vi "Catagorize VI.vi"(8 "error in (no error)":errorcluster {"code" format="Error %.0f"}, 10 "VI Reference":refnum<vi>, 11 "VIDoc Parser In":refnum<class "VIDoc Parser.lvclass">) -> (0 "error out":errorcluster {"code" format="Error %.0f"}, 3 "VIDoc Parser Out":refnum<class "VIDoc Parser.lvclass">)   [LabVIEW 2023, in "VIDoc Parsing.lvlib" / "VIDoc Parser.lvclass"]
uses:
  VIDoc Parser.lvclass
  VIDoc Parser.lvclass/VIDoc Parser.ctl
  <vilib>/Utility/lvfile.llb/NI_FileType.lvlib
  <vilib>/Utility/miscctls.llb/LVMapReplaceAction.ctl
  GUI Documentation/GUI Documentation.lvclass
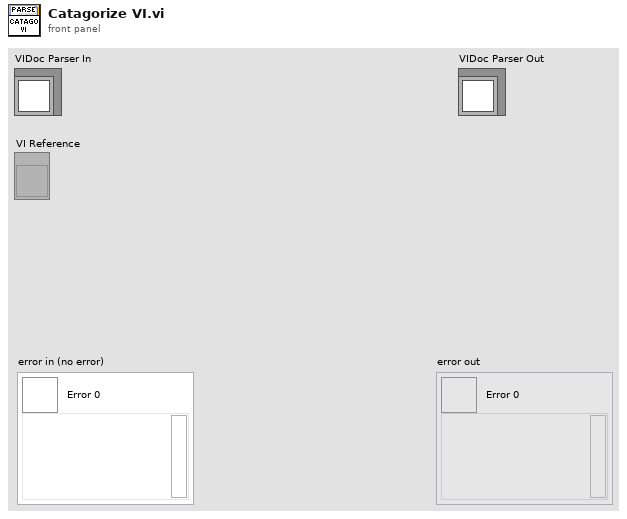
[diagram p1: front panel]
types:
  T1 = typedef "LVMapReplaceAction.ctl" = enum32{"Modify Entry only if found", "Add or Modify Entry", "Delete Entry"}
  T2 = typedef "NI_FileType.lvlib/FT_FileTypes.ctl" = enum32{"Invalid file/path", "Unknown type", "Instrument", "Control", "Polymorphic VI", "Project", "Library", "LVClass", "XControl", "XNode", "CIN", "Run-time menu", "Palette menu", "LLB", "Shortcut", "Directory", "Class Private Data Control", "Statechart", "MathScript .m file", "Ladder Diagram", "LVLibp"}
  T3 = enum32{"invalid VI type", "Standard VI", "Control VI", "Global VI", "Polymorphic VI", "Configuration VI", "SubSystem", "Facade VI", "Method VI", "Statechart Diagram VI"}
  T4 = typedef "VIDoc Parsing.lvlib/Parser Settings.lvclass/Parser Settings Cluster.ctl" = cluster{"Draw Controls":T5, "Max Control Recursion Depth":i32, "Bookmarks Map":map{string, string[]}}
  T5 = typedef "VIDoc Parsing.lvlib/Parser Settings.lvclass/Draw Controls Cluster.ctl" = cluster{"Subpanels":bool, "Tabs":bool, "TypeDefs":bool, "Error Clusters":T6, "DVRs":T6, "Queues & Notifiers":T6}
  T6 = typedef "VIDoc Parsing.lvlib/Parser Settings.lvclass/Draw Option Enum.ctl" = enum16{"Ignore", "Draw", "Draw + Contents"}
  T7 = map{string, refnum<class "GUI Documentation.lvclass">[]}
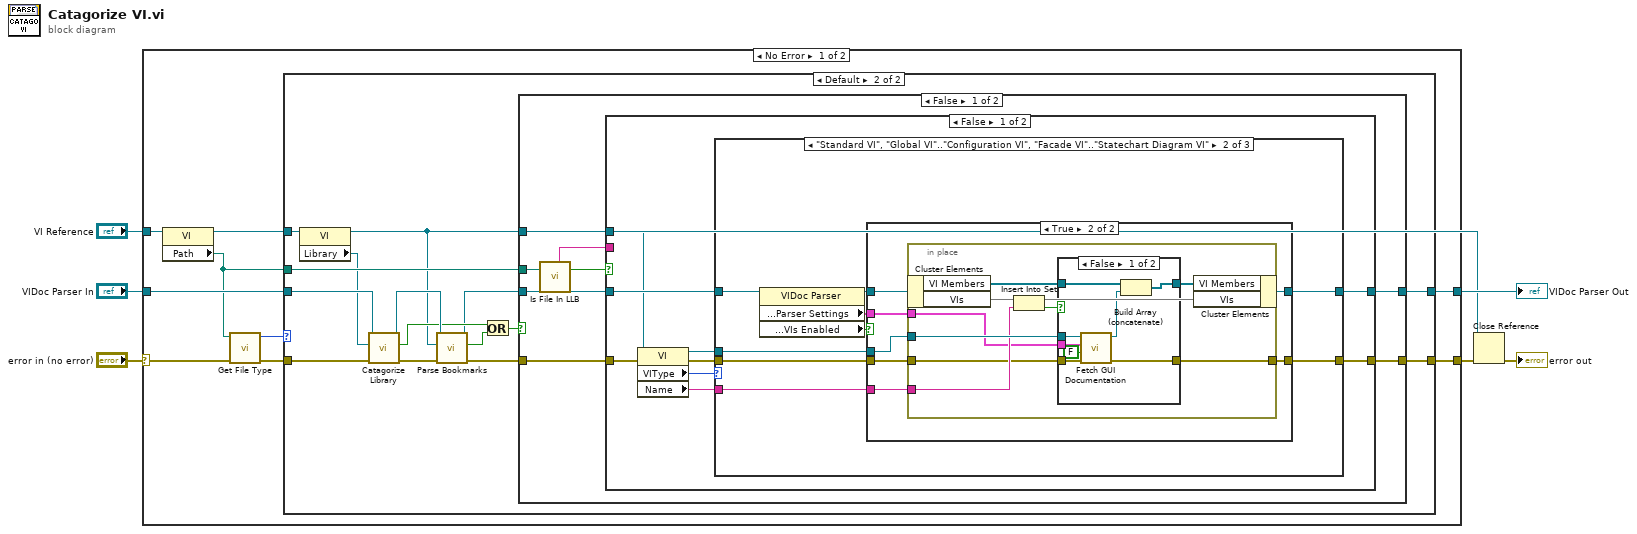
[diagram p0: block diagram]
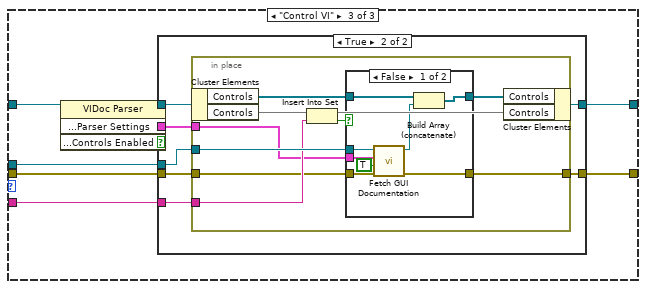
[diagram p6: hidden frame]
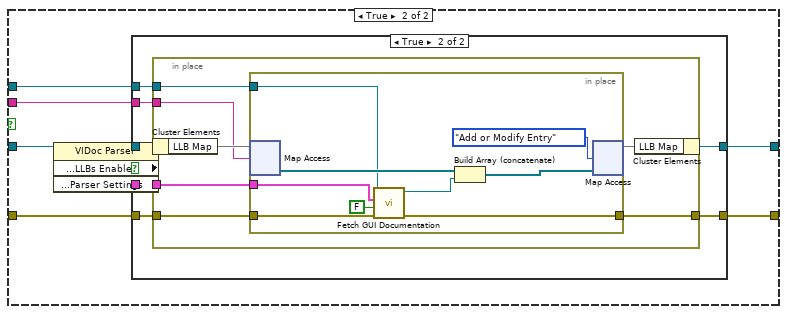
[diagram p9: hidden frame]
diagram:
  n1 = case shown="No Error" "error in (no error)" {
    selector: "error in (no error)" -> [w10 w165]
    tunnel: [w13 w165] -> w3
    tunnel: [w12 w164] -> w4
    tunnel: "VIDoc Parser In" -> [w14 w164]
    tunnel: "VI Reference" -> [w15 _]
    frame No Error {
      n2 = property class="VI"(reference=w15) -> (reference out=w11:refnum<vi>, "Path"=w7:path)  [unwired: 1 in, 1 out]
      n3 = call <vilib>:"Get File Type.vi"("error in (no error)"=w10, "path"=w7) -> ("error out"=w9:errorcluster, "file type"=w8:T2)  [unwired: 7 in, 1 out]
      n4 = case shown="Default" w8 {
        tunnel: w14 -> [w17 w32]
        tunnel: [w16 w19] -> w13
        tunnel: [w17 w26] -> w12
        tunnel: w11 -> [_ w25]
        tunnel: w9 -> [w16 w24]
        tunnel: w7 -> [_ w23]
        frame "Invalid file/path", "Class Private Data Control" {
        }
        frame Default {
          n5 = property class="VI"(reference=w25) -> (reference out=w22:refnum<vi>, "Library"=w21:refnum<vi>)  [unwired: 1 in, 1 out]
          n6 = call "Catagorize Library.vi"("error in (no error)"=w24, "Library"=w21, "VIDoc Parser In"=w32) -> ("error out"=w20:errorcluster, "Is Library?"=w29:bool, "VIDoc Parser Out"=w31:refnum<class "VIDoc Parser.lvclass">)  [unwired: 6 in]
          n7 = call "Parse Bookmarks.vi"("error in (no error)"=w20, "VI Reference"=w22, "VIDoc Parser In"=w31) -> ("error out"=w18:errorcluster, "Bookmarked?"=w30:bool, "VIDoc Parser Out"=w27:refnum<class "VIDoc Parser.lvclass">)  [unwired: 6 in]
          n8 = Or(x=w29, y=w30) -> (x .or. y?=w28:bool)
          n9 = case shown="False" w28 {
            tunnel: w18 -> [w40 w163]
            tunnel: [w39 w163] -> w19
            tunnel: w27 -> [w38 w162]
            tunnel: [w37 w162] -> w26
            tunnel: w22 -> [w36 _]
            tunnel: w23 -> [w35 _]
            frame False {
              n10 = call "Is File In LLB.vi"("Path"=w35) -> ("LLB Name"=w33:string, "Is in LLB?"=w34:bool)  [unwired: 5 in]
              n11 = case shown="False" w34 {
                tunnel: w40 -> [w49 w130]
                tunnel: [w41 w129] -> w39
                tunnel: w38 -> [w48 w136]
                tunnel: [w47 w135] -> w37
                tunnel: w36 -> [w46 w133]
                tunnel: w33 -> [_ w134]
                frame False {
                  n12 = property class="VI"(reference=w46, error in=w49) -> (reference out=w44:refnum<vi>, error out=w42:errorcluster, "VIType"=w45:T3, "Name"=w43:string)
                  n13 = case shown="\"Standard VI\", \"Global VI\"..\"Configuration VI\", \"Facade VI\"..\"Statechart Diagram VI\"" w45 {
                    tunnel: w44 -> [_ w57 w95]
                    tunnel: w48 -> [w51 w60 w98]
                    tunnel: [w51 w59 w97] -> w47
                    tunnel: w43 -> [_ w58 w96]
                    tunnel: w42 -> [w50 w56 w94]
                    tunnel: [w50 w55 w93] -> w41
                    frame Default {
                    }
                    frame "Standard VI", "Global VI".."Configuration VI", "Facade VI".."Statechart Diagram VI" {
                      n14 = property class="VIDoc Parser"(reference=w60) -> (reference out=w54:refnum<class "VIDoc Parser.lvclass">, "Properties:Settings:Parser Settings"=w52:T4, "Properties:Enabled:VIs Enabled"=w53:bool)  [unwired: 1 in, 1 out]
                      n15 = case shown="True" w53 {
                        tunnel: [w62 w69] -> w59
                        tunnel: w54 -> [w62 w68]
                        tunnel: w56 -> [w61 w67]
                        tunnel: [w61 w66] -> w55
                        tunnel: w52 -> [_ w65]
                        tunnel: w57 -> [_ w64]
                        tunnel: w58 -> [_ w63]
                        frame False {
                        }
                        frame True {
                          n16 = in-place "In Place Element Structure" {
                            in-place-border: w64 -> [w78]
                            in-place-border: w63 -> [w75]
                            in-place-border: w67 -> [w72]
                            in-place-border: [w71] -> w66
                            in-place-border: w65 -> [w70]
                            n17 = in-place-cluster #1(w68) -> ("VI Members"=w79:refnum<class "GUI Documentation.lvclass">[], "VIs"=w77:set{string})
                            n18 = Insert Into Set(10:w75, 11:w77) -> (2:w74:bool, 3:w76:set{string})
                            n19 = case shown="False" w74 {
                              tunnel: w79 -> [w87 w89]
                              tunnel: [w86 w89] -> w73
                              tunnel: w78 -> [w81 _]
                              tunnel: w72 -> [w85 w88]
                              tunnel: [w84 w88] -> w71
                              tunnel: w70 -> [w82 _]
                              frame False {
                                n20 = call "Fetch GUI Documentation.vi"("error in (no error)"=w85, "Fetch Controls?"=FALSE, "Parser Settings"=w82, "VI Reference"=w81) -> ("error out"=w84:errorcluster, "GUI Documentation Out"=w83:refnum<class "GUI Documentation.lvclass">)  [unwired: 6 in]
                                n21 = Build Array (concatenate)(w87, w83) -> (w86:refnum<class "GUI Documentation.lvclass">[])
                              }
                              frame True {
                              }
                            }
                            n22 = in-place-cluster #1("VI Members"=w73, "VIs"=w76) -> (w69:refnum<class "VIDoc Parser.lvclass">)
                          }
                        }
                      }
                    }
                    frame "Control VI" {
                      n23 = property class="VIDoc Parser"(reference=w98) -> (reference out=w92:refnum<class "VIDoc Parser.lvclass">, "Properties:Settings:Parser Settings"=w90:T4, "Properties:Enabled:Controls Enabled"=w91:bool)  [unwired: 1 in, 1 out]
                      n24 = case shown="True" w91 {
                        tunnel: [w100 w107] -> w97
                        tunnel: w92 -> [w100 w106]
                        tunnel: w94 -> [w99 w105]
                        tunnel: [w99 w104] -> w93
                        tunnel: w90 -> [_ w103]
                        tunnel: w95 -> [_ w102]
                        tunnel: w96 -> [_ w101]
                        frame False {
                        }
                        frame True {
                          n25 = in-place "In Place Element Structure" {
                            in-place-border: w102 -> [w116]
                            in-place-border: w101 -> [w113]
                            in-place-border: w105 -> [w110]
                            in-place-border: [w109] -> w104
                            in-place-border: w103 -> [w108]
                            n26 = in-place-cluster #2(w106) -> ("Controls"=w117:refnum<class "GUI Documentation.lvclass">[], "Controls"=w115:set{string})
                            n27 = Insert Into Set(10:w113, 11:w115) -> (2:w112:bool, 3:w114:set{string})
                            n28 = case shown="False" w112 {
                              tunnel: w117 -> [w125 w127]
                              tunnel: [w124 w127] -> w111
                              tunnel: w116 -> [w119 _]
                              tunnel: w110 -> [w123 w126]
                              tunnel: [w122 w126] -> w109
                              tunnel: w108 -> [w120 _]
                              frame False {
                                n29 = call "Fetch GUI Documentation.vi"("error in (no error)"=w123, "Fetch Controls?"=TRUE, "Parser Settings"=w120, "VI Reference"=w119) -> ("error out"=w122:errorcluster, "GUI Documentation Out"=w121:refnum<class "GUI Documentation.lvclass">)  [unwired: 6 in]
                                n30 = Build Array (concatenate)(w125, w121) -> (w124:refnum<class "GUI Documentation.lvclass">[])
                              }
                              frame True {
                              }
                            }
                            n31 = in-place-cluster #2("Controls"=w111, "Controls"=w114) -> (w107:refnum<class "VIDoc Parser.lvclass">)
                          }
                        }
                      }
                    }
                  }
                }
                frame True {
                  n32 = property class="VIDoc Parser"(reference=w136) -> (reference out=w132:refnum<class "VIDoc Parser.lvclass">, "Properties:Enabled:LLBs Enabled"=w131:bool, "Properties:Settings:Parser Settings"=w128:T4)  [unwired: 1 in, 1 out]
                  n33 = case shown="True" w131 {
                    tunnel: [w138 w145] -> w135
                    tunnel: w134 -> [_ w144]
                    tunnel: w133 -> [_ w143]
                    tunnel: w132 -> [w138 w142]
                    tunnel: w130 -> [w137 w141]
                    tunnel: [w137 w140] -> w129
                    tunnel: w128 -> [_ w139]
                    frame False {
                    }
                    frame True {
                      n34 = in-place "In Place Element Structure" {
                        in-place-border: w144 -> [w151]
                        in-place-border: w143 -> [w150]
                        in-place-border: w141 -> [w148]
                        in-place-border: [w147] -> w140
                        in-place-border: w139 -> [w146]
                        n35 = in-place-cluster #3(w142) -> ("LLB Map"=w152:T7)
                        n36 = in-place "In Place Element Structure" {
                          in-place-border: w150 -> [w158]
                          in-place-border: w148 -> [w156]
                          in-place-border: [w155] -> w147
                          in-place-border: w146 -> [w153]
                          n37 = in-place-map #4(w152, w151) -> (w161:refnum<class "GUI Documentation.lvclass">[])  [unwired: 1 in, 1 out]
                          n38 = call "Fetch GUI Documentation.vi"("error in (no error)"=w156, "Fetch Controls?"=FALSE, "Parser Settings"=w153, "VI Reference"=w158) -> ("error out"=w155:errorcluster, "GUI Documentation Out"=w157:refnum<class "GUI Documentation.lvclass">)  [unwired: 6 in]
                          n39 = Build Array (concatenate)(w161, w157) -> (w160:refnum<class "GUI Documentation.lvclass">[])
                          n40 = in-place-map #4(w160, LVMapReplaceAction."Add or Modify Entry" ("action")) -> (w149:T7)  [unwired: 2 out]
                        }
                        n41 = in-place-cluster #3("LLB Map"=w149) -> (w145:refnum<class "VIDoc Parser.lvclass">)
                      }
                    }
                  }
                }
              }
            }
            frame True {
            }
          }
        }
      }
    }
    frame Error {
    }
  }
  "VIDoc Parser Out" <- w4
  n42 = Close Reference(reference="VI Reference", error in (no error)=w3) -> (error out=→"error out":errorcluster)
